vi "DataLib.application example subscribe to event data.vi"() -> ()   [LabVIEW 2014, in "DataLib.lvlib"]
doc: "This is an example of a DIM client receiving service data via a message queue."
uses:
  DataLib.lvlib
  CS_Core/BaseProcess/BaseProcess.descriptor string definition.ctl
  CSlibraries-extern/DimLVEvent/LVDimInterface/LVDimInterface.dim service type.ctl
  CSlibraries-extern/DimLVEvent/LVDimInterface/LVDimInterface.dic_info_service_queue.vi
  CSlibraries-extern/DimLVEvent/LVDimInterface/LVDimInterface.lvlib
  CS_Core/BaseProcess/BaseProcess.lvlib
panel:
  out "subeventData":string[](array[string])
  out "dataDescriptors":T1[](array[typedef])
  out "dataObjects":string[](array[string])
  out "eventID":i32
  out "time stamp":timestamp
  out "headerID":timestamp
  out "error out":errorcluster
  out "no link":bool
  in  "serviceName":string="EventBuilder_eventData"
  out "receivedCounter":i32=1
  in  "stop":bool
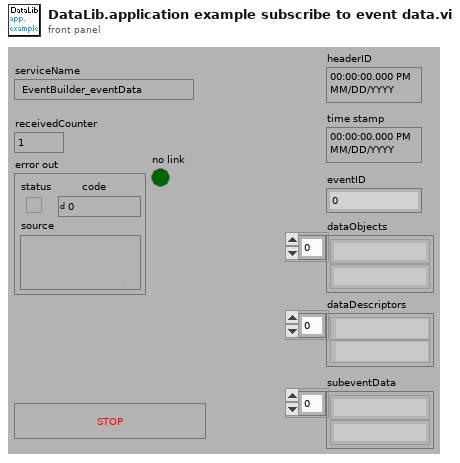
[diagram p1: front panel]
types:
  T1 = typedef "BaseProcess.lvlib/BaseProcess.descriptor string definition.ctl" = string
  T2 = typedef "LVDimInterface.lvlib/LVDimInterface.dim service type.ctl" = u16
  T3 = typedef "CoreDefs.rawDataType.ctl" = i8[]
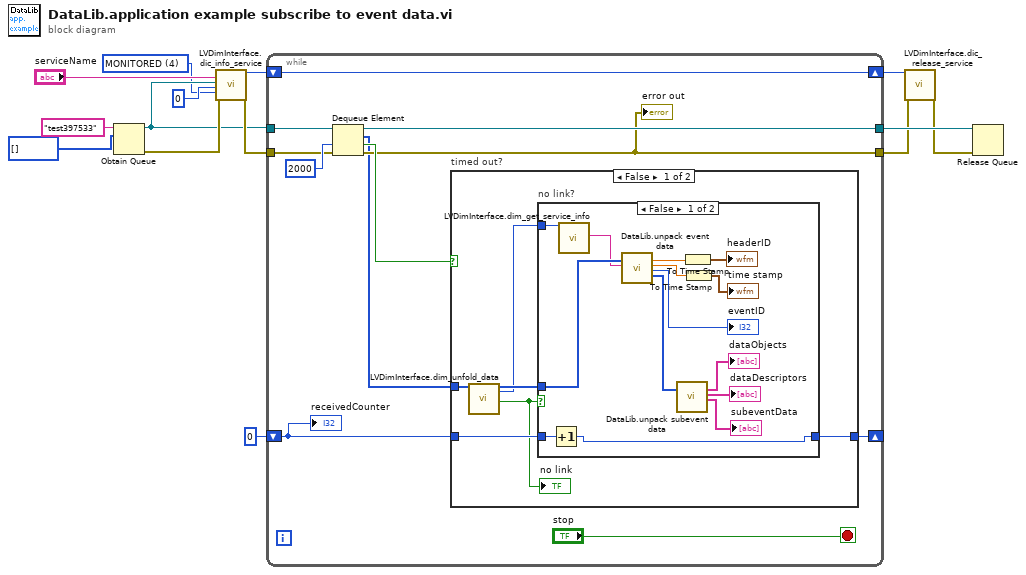
[diagram p0: block diagram]
diagram:
  w1 = T2 4 items=["ONCE_ONLY"=1, "TIMED"=2, "MONITORED"=4] ("serviceType")
  n1 = Obtain Queue(name (unnamed)="test397533", element data type=i8[] []) -> (queue out=w3:refnum<queue>, error out=w10:errorcluster)  [unwired: 3 in, 1 out]
  n2 = call-poly "LVDimInterface.dic_info_service.vi"("serviceName"="serviceName", "queueRef"=w3, "timeout [s]"=0, "serviceType"=w1, "error in (no error)"=w10) -> ("callBackID"=w13:i32, "error out"=w9:errorcluster)  [unwired: 13 in]
  n3 = while {
    tunnel: w3 -> [w25]
    tunnel: [w23] -> w12
    shift-right: [w19] -> _
    shift-left: 0 -> [w20]
    tunnel: w9 -> [w18]
    tunnel: [w17] -> w7
    shift-right: [w15] -> w8
    shift-left: w13 -> [w15]
    stop <- "stop" stop-if-true
    n4 = Dequeue Element(queue=w25, timeout in ms (-1)=2000, error in (no error)=w18) -> (queue out=w23:refnum<queue>, element=w16:i8[], timed out?=w22:bool, error out=w17:errorcluster)
    "error out" <- w17
    n5 = case "timed out?" shown="False" w22 {
      tunnel: [w30 w47] -> w19
      tunnel: w20 -> [w31 w47]
      tunnel: w16 -> [w28 _]
      frame False {
        n6 = call "LVDimInterface.dim_unfold_data.vi"("rawData"=w28) -> ("data"=w29:i8[], "callBackID"=w26:i32, "no link"=w27:bool)  [unwired: 15 in, 1 out]
        "no link" <- w27
        n7 = case "no link?" shown="False" w27 {
          tunnel: w31 -> [w45 w46]
          tunnel: [w44 w46] -> w30
          tunnel: w29 -> [w42 _]
          tunnel: w26 -> [w43 _]
          frame False {
            n8 = Increment(x=w45) -> (x+1=w44:i32)
            n9 = call "LVDimInterface.dim_get_service_info.vi"("callBackID"=w43) -> ("typeDescriptor"=w41:string)  [unwired: 9 in, 9 out]
            n10 = call "DataLib.unpack event data.vi"("serviceData"=w42, "descriptor"=w41) -> ("headerID"=w40:dbl, "timestamp"=w38:dbl, "eventID"=→"eventID":i32, "subEventData"=w35:T3)  [unwired: 13 in, 1 out]
            n11 = call "DataLib.unpack subevent data.vi"("subeventData"=w35) -> ("daqObjects"=→"dataObjects":string[], "dataDescriptors"=→"dataDescriptors":T1[], "subeventData"=→"subeventData":string[])  [unwired: 15 in, 1 out]
            n12 = To Time Stamp(1:w40) -> (0:→"headerID":timestamp)
            n13 = To Time Stamp(1:w38) -> (0:→"time stamp":timestamp)
          }
          frame True {
          }
        }
      }
      frame True {
      }
    }
    "receivedCounter" <- w20
  }
  n14 = call "LVDimInterface.dic_release_service.vi"("callBackID"=w8, "error in (no error)"=w7) -> ("error out"=w6:errorcluster)  [unwired: 17 in]
  n15 = Release Queue(queue=w12, error in (no error)=w6) -> ()  [unwired: 1 in, 3 out]
